vi "AnalogIO_ChannelLookup_Test.vi"() -> ()   [LabVIEW 2021]
uses:
  labbCAN_Bus_API/labbCAN_Bus_API.lvlib
  labbCAN_AnlogIO_API/labbCAN_AnalogIO_API.lvlib
panel:
  out "AnalogIn Channels":string[](array[string])
  out "Analog Input Count":i32
  out "AnalogOut Channels":string[](array[string])
  out "Analog Output Count":i32
  out "error out":errorcluster caption="Fehler (Ausgang)"
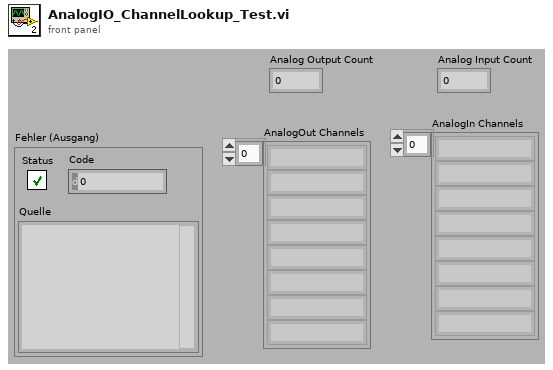
[diagram p1: front panel]
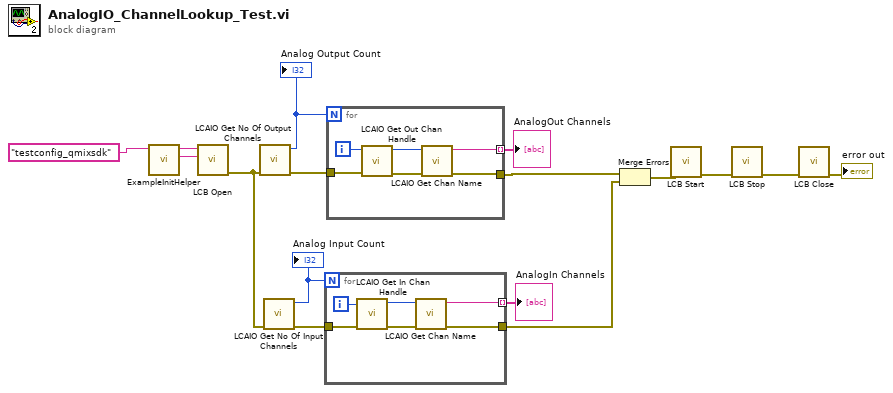
[diagram p0: block diagram]
diagram:
  n1 = call "ExampleInitHelper.vi"("Device Config Name"="testconfig_qmixsdk") -> ("Plugin Search Path"=w1:string, "Device Configuration Path"=w2:string)  [unwired: 5 in]
  n2 = call "LCB Open.vi"("PluginSearchPath"=w1, "Device Configuration Path"=w2) -> ("error out"=w10:errorcluster)  [unwired: 9 in]
  n3 = call "LCAIO Get No Of Output Channels.vi"("error in (no error)"=w10) -> ("error out"=w12:errorcluster, "Analog Output Count"=w13:i32)  [unwired: 9 in]
  "Analog Output Count" <- w13
  n4 = call "LCAIO Get No Of Input Channels.vi"("error in (no error)"=w10) -> ("error out"=w9:errorcluster, "Analog Input Count"=w8:i32)  [unwired: 9 in]
  "Analog Input Count" <- w8
  n5 = for {
    N: w8 -> [_]
    tunnel: w9 -> [w22]
    tunnel: [w19] -> w5
    tunnel: [w18] -> w7 mode=indexing
    i -> [w17]
    n6 = call "LCAIO Get In Chan Handle.vi"("error in (no error)"=w22, "Index"=w17) -> ("error out"=w21:errorcluster, "Analog Input"=w20:i64)  [unwired: 8 in]
    n7 = call "LCAIO Get Chan Name.vi"("error in (no error)"=w21, "Channel Handle"=w20) -> ("error out"=w19:errorcluster, "Name"=w18:string)  [unwired: 8 in]
  }
  "AnalogIn Channels" <- w7
  n8 = for {
    N: w13 -> [_]
    tunnel: [w24] -> w6
    tunnel: w12 -> [w27]
    tunnel: [w23] -> w11 mode=indexing
    i -> [w28]
    n9 = call "LCAIO Get Out Chan Handle.vi"("error in (no error)"=w27, "Index"=w28) -> ("error out"=w26:errorcluster, "Analog Output Channel"=w25:i64)  [unwired: 8 in]
    n10 = call "LCAIO Get Chan Name.vi"("error in (no error)"=w26, "Channel Handle"=w25) -> ("error out"=w24:errorcluster, "Name"=w23:string)  [unwired: 8 in]
  }
  "AnalogOut Channels" <- w11
  n11 = Merge Errors(w6, w5) -> (w4:errorcluster)
  n12 = call "LCB Start.vi"("error in (no error)"=w4) -> ("error out"=w14:errorcluster)  [unwired: 10 in]
  n13 = call "LCB Stop.vi"("error in (no error)"=w14) -> ("error out"=w15:errorcluster)  [unwired: 10 in]
  n14 = call "LCB Close.vi"("error in (no error)"=w15) -> ("error out"=→"error out":errorcluster)  [unwired: 10 in]
